vi "play_sysID_Z_Axis_simple.vi"() -> ()   [LabVIEW 2017]
uses:
  sysID_Z-axis-params.ctl
  <vilib>/FPGAPlugInAG/cRIO-9082/niLvFpga_Open_cRIO-9082.vi
  <vilib>/rvi/interface/common/dynamic/niFpgaDynamicAddResources.vi
  <vilib>/FPGAPlugInAG/Dynamic/niLvFpga_Reset_Dynamic.vi
  <vilib>/rvi/interface/common/niFpgaWaitOnOcc.vi
  <vilib>/Utility/error.llb/Error Cluster From Error Code.vi
  <vilib>/rvi/errors/niLvFpgaAdjustHostInterfaceError.vi
  <vilib>/FPGAPlugInAG/Dynamic/niLvFpga_Run_Dynamic.vi
  <vilib>/FPGAPlugInAG/Dynamic/niLvFpga_Close_Dynamic.vi
  <vilib>/rvi/interface/nirviOpenFPGA/nirviOpenFPGA.xnode
  FPGA Bitfiles/afmimagingcontro_FPGATargetSPARTA_fpgasysIDZaxissi_jhd3Wt3fyx0.lvbitx
  <vilib>/rvi/interface/nirviMethod/nirviMethod.xnode
  <vilib>/rvi/interface/nirviReadWriteControl/nirviReadWriteControl.xnode
  <vilib>/rvi/interface/nirviCloseFPGA/nirviCloseFPGA.xnode
  <vilib>/FPGAPlugInAG/Dynamic/niLvFpga_ConfigureFifo_Dynamic.vi
  <vilib>/rvi/errors/niLvFpgaMergeErrorWithErrorCode.vi
  NiFpgaLv.dll
  <vilib>/rvi/interface/Simulation/niFpgaSimulationCallBeginRW.vi
panel:
  out "input fifo num":i16
  out "log fifo num":i16
  out "logging-timeout?":bool
  out "Current Case":i16
  in  "ABORT":bool
  in  "Cluster":T1={"TOL"=0.3, "ramp-rate"=-5e-06, "z-u-max"=5.0, "offset"=0.0, "Ki"=0.001, "Z-error-threshold"=0.2, "Z-settled-samples\nthreshold "=200, "z_UP"=1.5, "zup-N"=5000} {"Z-error-threshold" format="%#_13g"; "ramp-rate" format="%#_4g"; "TOL" format="%#_13g"}
  in  "Z up":fxp<+/-,16,5>
  in  "trigger-0":bool
  out "boolean  indicators 2":T2
  out "dataIn Path":path
  out "uzk)":dbl[](graph)
  out "z-err(k)":dbl[](graph)
  out "size(s)":i32
  out "Nsamps_i":i32
  out "error":errorcluster
  in  "expName (e.g. 25-Mar-2106_exp001)":string="10-Aug-2017_exp01_multiAxis"
  out "Current Freq":dbl format="%#_13g"
  out "freqs":dbl[](array[numeric])
  out "Elements Remaining":i32=1
  out "ref(k) Signal":dbl[](graph)
  in  "Input Folder":path=path "C:/Users/arnold/Documents/MATLAB/AFM_SS/System_Identification/data/data_ZAxis"
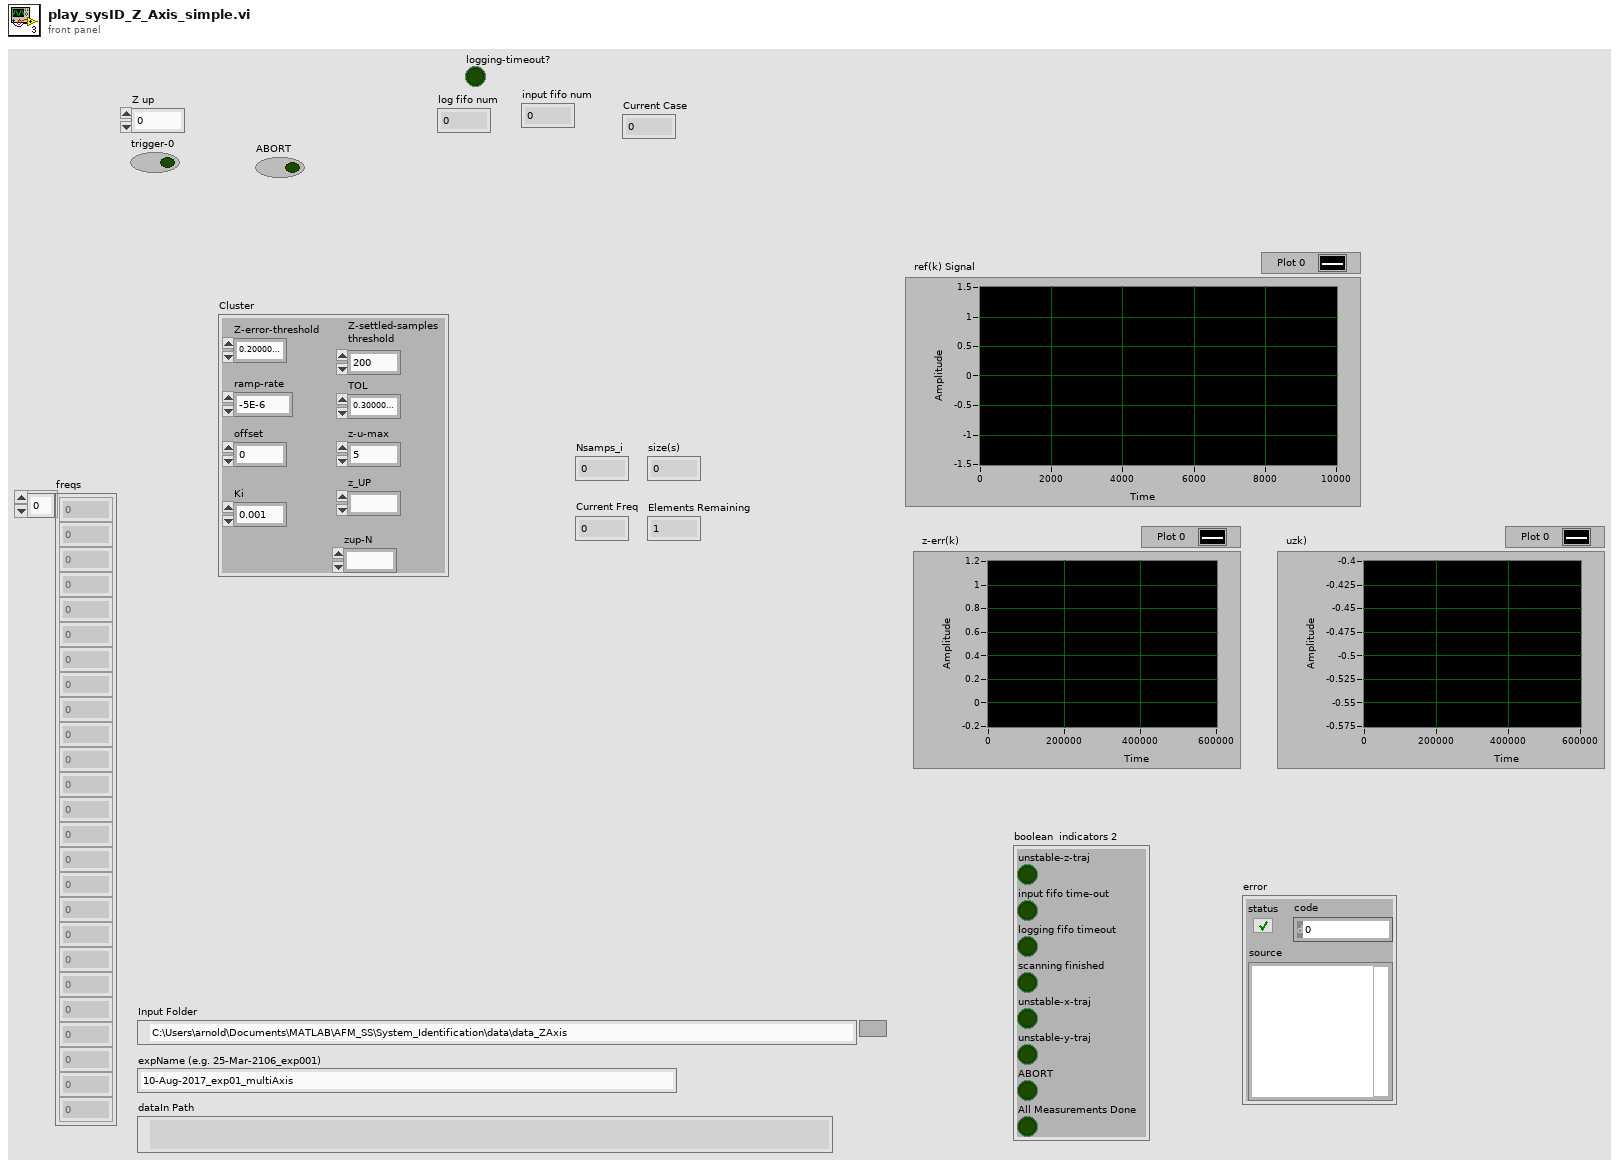
[diagram p1: front panel]
types:
  T1 = typedef "sysID_Z-axis-params.ctl" = cluster{"TOL":sgl, "ramp-rate":sgl, "z-u-max":sgl, "offset":sgl, "Ki":sgl, "Z-error-threshold":sgl, "Z-settled-samples\nthreshold ":i16, "z_UP":fxp<+/-,16,5>, "zup-N":i16}
  T2 = cluster{"unstable-z-traj":bool, "input fifo time-out":bool, "logging fifo timeout":bool, "scanning finished":bool, "unstable-x-traj":bool, "unstable-y-traj":bool, "ABORT":bool, "All Measurements Done":bool}
  T3 = typedef "sysID_ControlParams.ctl" = cluster{"Kp":sgl, "Umax ":sgl, "ymax":sgl, "TsTicks":u32, "z1":sgl, "num":sgl[], "den":sgl[], "TF Order":u8}
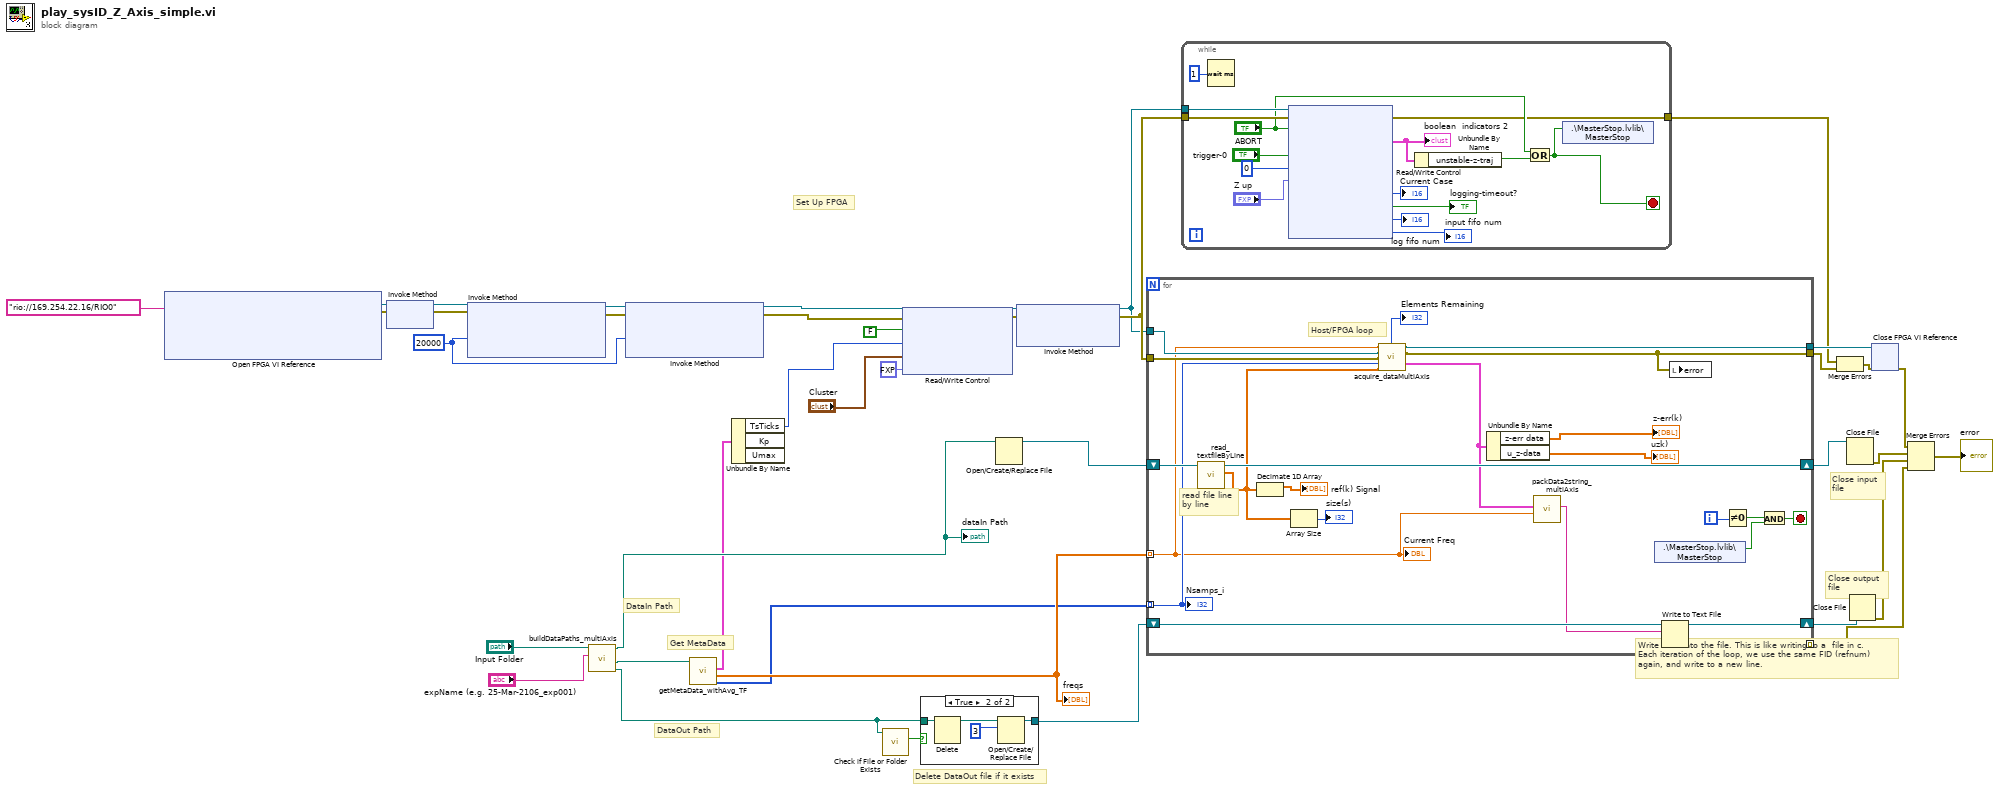
[diagram p0: block diagram]
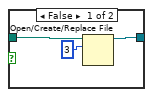
[diagram p2: hidden frame]
diagram:
  w5 = 20000 ("requested depth")
  # "Set Up FPGA"
  # "Delete DataOut file if it exists"
  # "Close output\nfile"
  # "Close input\nfile"
  # "Write data into the file. This is like writing to a  file in c.\nEach iteration of the loop, we use the same FID (refnum) \nagain, and write to a new line."
  # "DataIn Path"
  # "DataOut Path"
  # "Get MetaData"
  n1 = xnode "Open FPGA VI Reference"("resource name"=tag "rio://169.254.22.16/RIO0") -> ("FPGA VI Reference Out"=w14:refnum<k20>, "error out"=w13:errorcluster)  [unwired: 1 in]
  n2 = xnode "Invoke Method"("FPGA VI Reference In"=w14, "error in"=w13) -> ("FPGA VI Reference Out"=w18:refnum<k20>, "error out"=w17:errorcluster)
  n3 = xnode "Invoke Method"("FPGA VI Reference In"=w18, "error in"=w17, "Requested Depth"=w5) -> ("FPGA VI Reference Out"=w16:refnum<k20>, "error out"=w15:errorcluster)  [unwired: 1 out]
  n4 = call "buildDataPaths_multiAxis.vi"("expName"="expName (e.g. 25-Mar-2106_exp001)", "Data Folder"="Input Folder") -> ("dataOut path"=w20:path, "metaData Path"=w25:path, "dataIn Path"=w26:path)  [unwired: 7 in]
  "dataIn Path" <- w26
  n5 = xnode "Invoke Method"("FPGA VI Reference In"=w16, "error in"=w15, "Requested Depth"=w5) -> ("FPGA VI Reference Out"=w12:refnum<k20>, "error out"=w11:errorcluster)  [unwired: 1 out]
  n6 = call "getMetaData_withAvg_TF.vi"("MetaDataPath"=w25) -> ("Num Samples"=w27:i32[], "freqs (hz)"=w28:dbl[], "ControlParams"=w10:T3)  [unwired: 7 in]
  "freqs" <- w28
  n7 = Unbundle By Name(w10) -> ("TsTicks"=w6:u32)  [unwired: 2 out]
  n8 = call <vilib>:"Check if File or Folder Exists.vi"("path"=w20) -> ("file or folder exists?"=w19:bool)  [unwired: 8 in, 2 out]
  n9 = xnode "Read/Write Control"("FPGA VI Reference In"=w12, "error in"=w11, "ABORT"=FALSE, "TsTicks"=w6, "sysID_Z_axis_params"="Cluster", "init Z up"=fxp<+/-,16,5> 0.0) -> ("FPGA VI Reference Out"=w39:refnum<k20>, "error out"=w40:errorcluster)
  n10 = case shown="True" w19 {
    tunnel: w20 -> [w42 w47]
    tunnel: [w41 w45] -> w29
    frame False {
      n11 = Open/Create/Replace File(file path (use dialog)=w42, operation (0:open)=3) -> (refnum out=w41:refnum<file>)  [unwired: 4 in, 2 out]
    }
    frame True {
      n12 = Delete(path (use dialog)=w47) -> (deleted path=w46:path)  [unwired: 4 in, 2 out]
      n13 = Open/Create/Replace File(file path (use dialog)=w46, operation (0:open)=3) -> (refnum out=w45:refnum<file>)  [unwired: 4 in, 2 out]
    }
  }
  n14 = Open/Create/Replace File(file path (use dialog)=w26) -> (refnum out=w35:refnum<file>)  [unwired: 5 in, 2 out]
  n15 = xnode "Invoke Method"("FPGA VI Reference In"=w39, "error in"=w40) -> ("FPGA VI Reference Out"=w8:refnum<k20>, "error out"=w9:errorcluster)  [unwired: 1 in]
  n16 = for {
    tunnel: [w63] -> w38
    tunnel: [w52] -> w1
    tunnel: w9 -> [w60]
    tunnel: w8 -> [w62]
    tunnel: w28 -> [w58] mode=indexing
    shift-right: [w70] -> w37
    shift-left: w29 -> [w69]
    shift-right: [w68] -> w36
    shift-left: w35 -> [w67]
    tunnel: w27 -> [w61] mode=indexing
    tunnel: [w65] -> w30 mode=indexing
    i -> [w51]
    stop <- w48 stop-if-true
    # "Host/FPGA loop"
    # "read file line\nby line"
    n17 = call "read_textfileByLine.vi"("Byte Stream File in"=w67) -> ("Array"=w53:dbl[], "Byte Stream File out"=w68:refnum<file>)  [unwired: 9 in]
    n18 = Decimate 1D Array(w53) -> (→"ref(k) Signal":dbl[])  [unwired: 1 out]
    n19 = Array Size(array=w53) -> (size(s)=→"size(s)":i32)
    n20 = call "acquire_dataMultiAxis.vi"("Freq_i"=w58, "FPGA VI Reference in"=w62, "error in"=w60, "Nsamps_i"=w61, "data (sin wave) in"=w53) -> ("Elements Remaining"=→"Elements Remaining":i32, "FPGA VI Reference Out"=w63:refnum<k20>, "error IO"=w52:errorcluster, "output cluster"=w57:cluster{"z-err data":dbl[], "u_z-data":dbl[]})  [unwired: 6 in, 1 out]
    n21 = Unbundle By Name(w57) -> ("z-err data"=→"z-err(k)":dbl[], "u_z-data"=→"uzk)":dbl[])
    n22 = call "packData2string_multiAxis.vi"("F_i: current freq"=w58, "output cluster"=w57) -> ("spreadsheet string"=w59:string)  [unwired: 9 in]
    n23 = shared-variable ".\\MasterStop.lvlib\\MasterStop"() -> (w49:bool)  [unwired: 1 in, 1 out]
    n24 = Write to Text File(file (use dialog)=w69, text=w59) -> (refnum out=w70:refnum<file>, error out=w65:errorcluster)  [unwired: 2 in, 1 out]
    n25 = local write "error"(w52) -> ()
    n26 = Not Equal To 0?(x=w51) -> (x != 0?=w50:bool)
    n27 = And(x=w50, y=w49) -> (x .and. y?=w48:bool)
    "Current Freq" <- w58
    "Nsamps_i" <- w61
  }
  n28 = while {
    tunnel: w8 -> [w84]
    tunnel: w9 -> [w83]
    tunnel: [w71] -> w2
    stop <- w76 stop-if-true
    n29 = Wait (ms)(milliseconds to wait=u32 1) -> ()  [unwired: 1 out]
    n30 = xnode "Read/Write Control"("FPGA VI Reference In"=w84, "error in"=w83, "ABORT"="ABORT", "trigger-0"="trigger-0", "initial case"=i16 0, "init Z up"="Z up") -> ("error out"=w71:errorcluster, "boolean  indicators"=w79:T2, "Current Case"=→"Current Case":i16, "logging-timeout?"=→"logging-timeout?":bool, "Numeric"=→"log fifo num":u32, "Numeric 2"=→"input fifo num":u32)  [unwired: 1 out]
    "boolean  indicators 2" <- w79
    n31 = Unbundle By Name(w79) -> ("unstable-z-traj"=w78:bool)
    n32 = Or(x="ABORT", y=w78) -> (x .or. y?=w76:bool)
    n33 = shared-variable ".\\MasterStop.lvlib\\MasterStop"(w76) -> ()  [unwired: 1 in, 1 out]
  }
  n34 = Merge Errors(w2, w1) -> (w3:errorcluster)
  n35 = Close File(refnum=w36) -> (error out=w33:errorcluster)  [unwired: 1 in, 1 out]
  n36 = Close File(refnum=w37) -> (error out=w34:errorcluster)  [unwired: 1 in, 1 out]
  n37 = xnode "Close FPGA VI Reference"("FPGA VI Reference In"=w38, "error in"=w3) -> ("error out"=w31:errorcluster)
  n38 = Merge Errors(w31, w33, w34, w30) -> (→"error":errorcluster)
